vi "CheckPosCon.vi"(9 "Sequential Checks":dbl, 10 "WasRight":bool) -> (2 "We made It":bool)   [LabVIEW 2020]
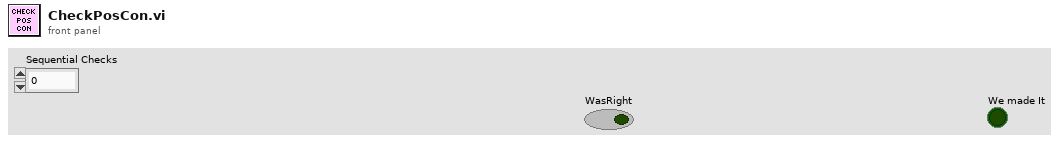
[diagram p1: front panel]
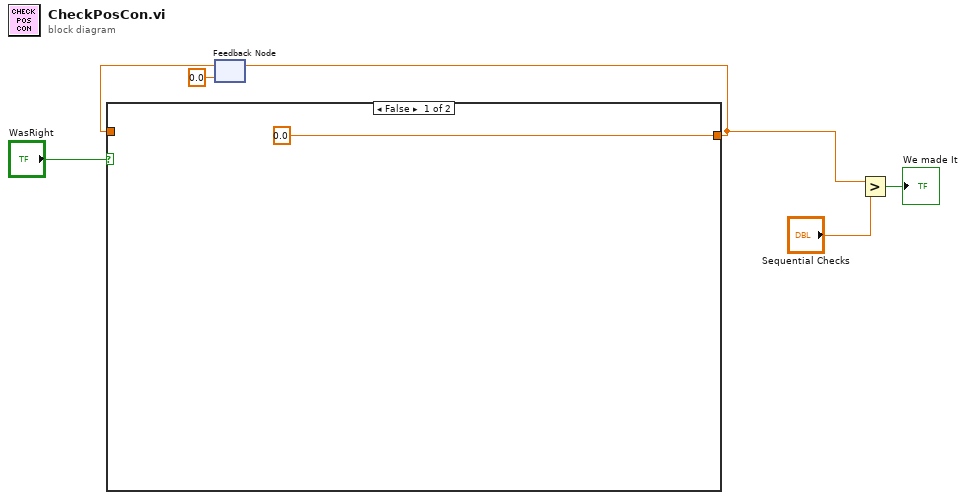
[diagram p0: block diagram]
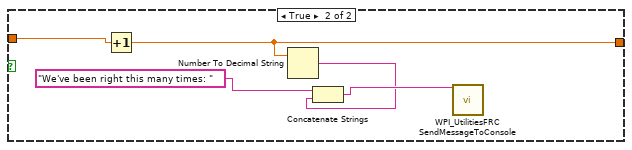
[diagram p2: hidden frame]
diagram:
  n1 = feedback #1(0.0) -> (w6:dbl)
  n2 = case shown="False" "WasRight" {
    tunnel: w6 -> [_ w12]
    tunnel: [0.0 w11] -> w4
    frame False {
    }
    frame True {
      n3 = Increment(x=w12) -> (x+1=w11:dbl)
      n4 = Number To Decimal String(number=w11) -> (decimal integer string=w8:string)  [unwired: 1 in]
      n5 = Concatenate Strings("We've been right this many times: ", w8) -> (w10:string)
      n6 = call <vilib>:"WPI_UtilitiesFRC SendMessageToConsole.vi"("Message"=w10) -> ()  [unwired: 14 in, 1 out]
    }
  }
  n7 = feedback-in #1(w4) -> ()
  n8 = Greater?(x=w4, y="Sequential Checks") -> (0:→"We made It":bool)
